vi "LeCroy.Self-Test.vi"(8 "Error In":errorcluster, 11 "LeCroy.Session in":T1) -> (0 "Error Out":errorcluster, 2 "Self-Test Result Code":i32, 3 "LeCroy.Session out":T1)   [LabVIEW 2018]
uses:
  typedefs/LeCroy.Session.ctl
  <instrlib>/LeCroy Wave Series/LeCroy Wave Series.lvlib
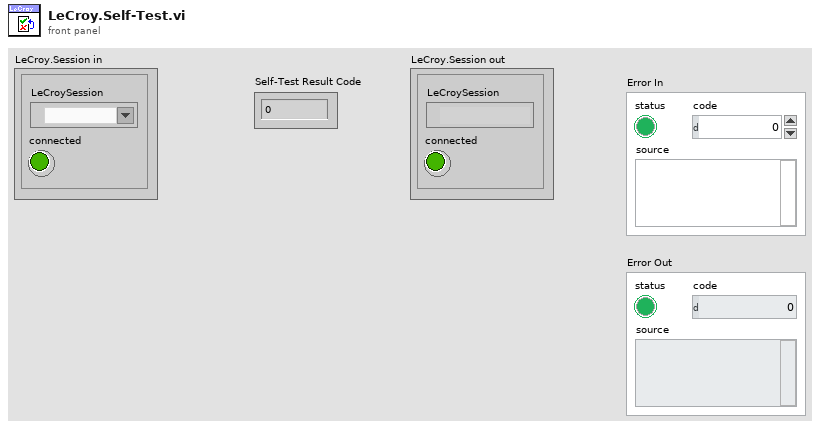
[diagram p1: front panel]
types:
  T1 = typedef "LeCroy.Session.ctl" = cluster{"LeCroySession":refnum<visa-resource-name>, "connected":bool}
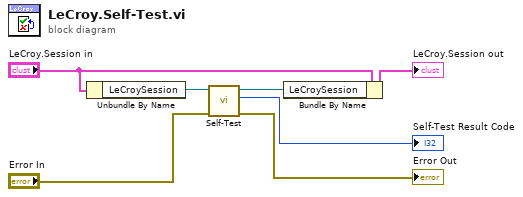
[diagram p0: block diagram]
diagram:
  n1 = Unbundle By Name("LeCroy.Session in") -> ("LeCroySession"=w7:refnum<visa-resource-name>)
  n2 = call <instrlib>:"Self-Test.vi"("error in (no error)"="Error In", "VISA resource name"=w7) -> ("error out"=→"Error Out":errorcluster, "Self-Test Result Code"=→"Self-Test Result Code":i32, "VISA resource name out"=w4:refnum<visa-resource-name>)  [unwired: 6 in, 1 out]
  n3 = Bundle By Name(cluster="LeCroy.Session in", "LeCroySession"=w4) -> (→"LeCroy.Session out":T1)
